vi "Poll Until Idle.vi"(8 "error in (no error)":errorcluster, 9 "Device and Axis":string, 11 "VISA resource name":refnum<visa-resource-name>) -> (0 "error out":errorcluster, 3 "VISA resource name out":refnum<visa-resource-name>)   [LabVIEW 2020, in "Zaber A Series.lvlib"]
doc: "Waits for any movement of the device to complete and the device to be idle before continuing. To poll a specific device, use the Device and Axis input. This VI is not designed to poll all devices unless only one device is connected.\n\nTo avoid saturating the CPU or the communication channel, this VI will poll once every 25ms. There is no wait if the device is in the idle state.\n\nThis VI requires that the Initialize VI has been called with the same serial port."
uses:
  Zaber A Series.lvlib
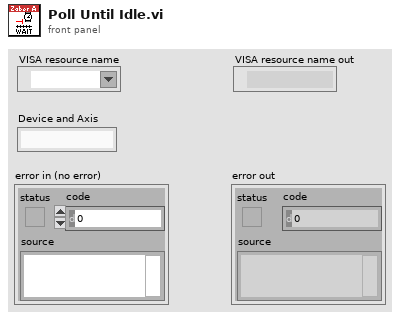
[diagram p1: front panel]
types:
  T1 = cluster{"Device":string, "Axis":string, "Reply Flag":string, "Status":string, "Warning Flags":string, "Data":string}[]
  T2 = cluster{"Device":string, "Axis":string, "Reply Flag":string, "Status":string, "Warning Flags":string, "Data":string}
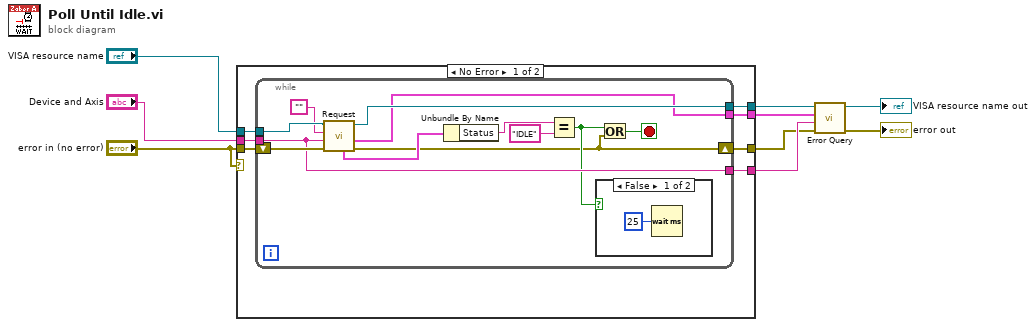
[diagram p0: block diagram]
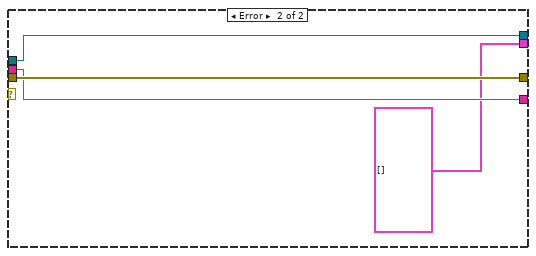
[diagram p3: hidden frame]
diagram:
  n1 = case shown="No Error" "error in (no error)" {
    tunnel: "VISA resource name" -> [w16 w31]
    tunnel: "error in (no error)" -> [w15 w33]
    tunnel: "Device and Axis" -> [w14 w32]
    tunnel: [w13 w32] -> w7
    tunnel: [w12 T1 [] ("Response Bundle Array")] -> w6
    tunnel: [w11 w31] -> w5
    tunnel: [w10 w33] -> w3
    frame No Error {
      n2 = while {
        tunnel: w16 -> [w26]
        tunnel: [w25] -> w11
        tunnel: w14 -> [w22]
        shift-right: [w17] -> w10
        shift-left: w15 -> [w24]
        tunnel: [w20] -> w12
        tunnel: [w22] -> w13
        stop <- w19 stop-if-true
        n3 = call "Request.vi"("error in (no error)"=w24, "Device and Axis"=w22, "Command String"="", "VISA resource name"=w26) -> ("error out"=w17:errorcluster, "Response Bundle Array"=w20:T1, "VISA resource name out"=w25:refnum<visa-resource-name>, "First Response Bundle"=w21:T2)  [unwired: 2 in, 2 out]
        n4 = Unbundle By Name(w21) -> ("Status"=w27:string)
        n5 = Equal?(x=w27, y="IDLE") -> (x = y?=w18:bool)
        n6 = case shown="False" w18 {
          frame False {
            n7 = Wait (ms)(milliseconds to wait=u32 25) -> ()  [unwired: 1 out]
          }
          frame True {
          }
        }
        n8 = Or(x=w18, y=w17) -> (x .or. y?=w19:bool)
      }
    }
    frame Error {
    }
  }
  n9 = call "Error Query.vi"("error in (no error)"=w3, "Device and Axis"=w7, "Previous Response Bundle Array"=w6, "VISA resource name"=w5) -> ("error out"=→"error out":errorcluster, "VISA resource name out"=→"VISA resource name out":refnum<visa-resource-name>)  [unwired: 4 in, 2 out]
